vi "Set Exp Param and Set Delays.vi"(0 "Control-Client in":refnum<class "Control-Client.lvclass">, 5 "remake":bool, 11 "error in (no error)":errorcluster) -> (4 "Control-Client out":refnum<class "Control-Client.lvclass">, 15 "error out":errorcluster)   [LabVIEW 2018, in "Control-Client.lvclass"]
uses:
  Control-Client.lvclass
  Control-Client.lvclass/Control-Client.ctl
  Experiments/Experiment.lvclass/Experiment.ctl
  Experiments/Experiment.lvclass
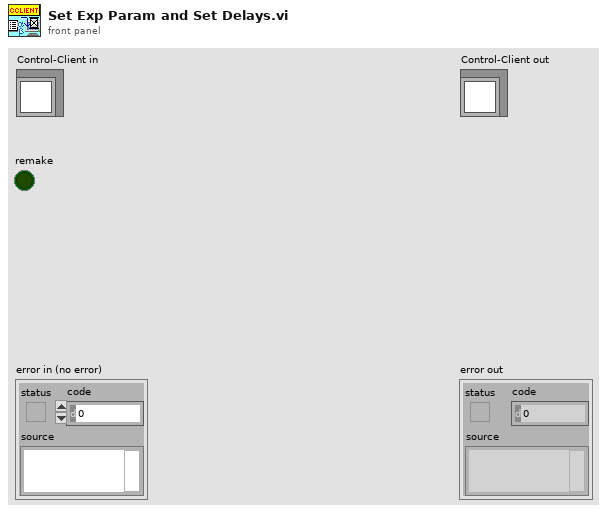
[diagram p1: front panel]
types:
  T1 = typedef "Control-Client.lvclass/Delays-refs_CLIENT.ctl" = cluster{"# points":refnum<vi>, "Step, ps":refnum<vi>, "OZ, ps":refnum<vi>, "# current":refnum<vi>, "RDT, ps":refnum<vi>, "Total length, ps":refnum<vi>, "Kinetics length, ps":refnum<vi>, "Real zero, ps":refnum<vi>, "# par point":refnum<vi>}
  T2 = cluster{"min I, mm":dbl, "max I, mm":dbl, "Real Optical 0, ps":dbl, "min II, mm":dbl, "max II, mm ":dbl}
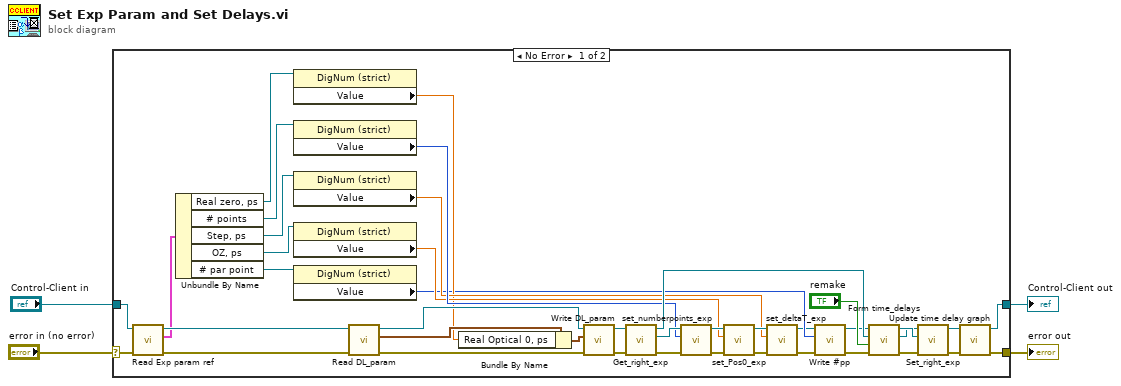
[diagram p0: block diagram]
diagram:
  n1 = case shown="No Error" "error in (no error)" {
    selector: "error in (no error)" -> [w42 w46]
    tunnel: [w18 w46] -> w3
    tunnel: [w19 w45] -> w1
    tunnel: "Control-Client in" -> [w44 w45]
    frame No Error {
      n2 = call "Read Exp param ref.vi"("error in (no error)"=w42, "Control-Client in"=w44) -> ("error out"=w41:errorcluster, "Exp param ref"=w40:T1, "Control-Client out"=w43:refnum<class "Control-Client.lvclass">)  [unwired: 7 in]
      n3 = Unbundle By Name(w40) -> ("Real zero, ps"=w39:refnum<vi>, "# points"=w36:refnum<vi>, "Step, ps"=w37:refnum<vi>, "OZ, ps"=w38:refnum<vi>, "# par point"=w10:refnum<vi>)
      n4 = property class="DigNum (strict)"(reference=w39) -> ("Value"=w15:dbl)  [unwired: 1 in, 2 out]
      n5 = property class="DigNum (strict)"(reference=w36) -> ("Value"=w23:i32)  [unwired: 1 in, 2 out]
      n6 = property class="DigNum (strict)"(reference=w37) -> ("Value"=w22:dbl)  [unwired: 1 in, 2 out]
      n7 = property class="DigNum (strict)"(reference=w38) -> ("Value"=w21:dbl)  [unwired: 1 in, 2 out]
      n8 = property class="DigNum (strict)"(reference=w10) -> ("Value"=w9:i32)  [unwired: 1 in, 2 out]
      n9 = call "Read DL_param.vi"("error in (no error)"=w41, "Control-Client in"=w43) -> ("error out"=w34:errorcluster, "DL_param"=w33:T2, "Control-Client out"=w35:refnum<class "Control-Client.lvclass">)  [unwired: 7 in]
      n10 = Bundle By Name(cluster=w33, "Real Optical 0, ps"=w15) -> (w32:T2)
      n11 = call "Write DL_param.vi"("error in (no error)"=w34, "DL_param"=w32, "Control-Client in"=w35) -> ("error out"=w14:errorcluster, "Control-Client out"=w13:refnum<class "Control-Client.lvclass">)  [unwired: 7 in]
      n12 = call "Get_right_exp.vi"("error in (no error)"=w14, "Control-Client in"=w13) -> ("error out"=w28:errorcluster, "Right experiment"=w29:refnum<class "Experiment.lvclass">, "Control-Client out"=w30:refnum<class "Control-Client.lvclass">)  [unwired: 7 in]
      n13 = call "set_numberpoints_exp.vi"("error in (no error)"=w28, "numberpoints"=w23, "Experiment.lvclass in"=w29) -> ("error out"=w27:errorcluster, "Experiment.lvclass out"=w24:refnum<class "Experiment.lvclass">)  [unwired: 6 in]
      n14 = call "set_Pos0_exp.vi"("error in (no error)"=w27, "Pos0,ps"=w21, "Experiment.lvclass in"=w24) -> ("error out"=w26:errorcluster, "Experiment.lvclass out"=w25:refnum<class "Experiment.lvclass">)  [unwired: 6 in]
      n15 = call "set_deltaT_exp.vi"("error in (no error)"=w26, "deltaTlast"=w22, "Experiment.lvclass in"=w25) -> ("error out"=w5:errorcluster, "Experiment.lvclass out"=w8:refnum<class "Experiment.lvclass">)  [unwired: 6 in]
      n16 = call "Write #pp.vi"("error in (no error)"=w5, "#pp"=w9, "Experiment in"=w8) -> ("error out"=w6:errorcluster, "Experiment out"=w7:refnum<class "Experiment.lvclass">)  [unwired: 7 in]
      n17 = call "Form time_delays.vi"("error in (no error)"=w6, "remake"="remake", "Control-Client"=w30, "Experiment in"=w7) -> ("error out"=w12:errorcluster, "Control-Client out"=w11:refnum<class "Control-Client.lvclass">, "Experiment out"=w31:refnum<class "Experiment.lvclass">)  [unwired: 5 in]
      n18 = call "Set_right_exp.vi"("error in (no error)"=w12, "Experiment in"=w31, "Control-Client in"=w11) -> ("error out"=w17:errorcluster, "Control-Client out"=w20:refnum<class "Control-Client.lvclass">)  [unwired: 7 in]
      n19 = call "Update time delay graph.vi"("error in (no error)"=w17, "Control-Client en entrée"=w20) -> ("error out"=w18:errorcluster, "Control-Client en sortie"=w19:refnum<class "Control-Client.lvclass">)  [unwired: 8 in]
    }
    frame Error {
    }
  }
  "error out" <- w3
  "Control-Client out" <- w1
